vi "USERCallVISample.vi"(4 "Thread No.":u32, 5 "ProgramRef":refnum<vi>, 6 "Thread Mod Recive":refnum<queue>[](array[refnum]), 7 "ThreadsQueue":refnum<queue>[](array[refnum]), 8 "ThreadInfoIN":T1, 10 "StackIn":cluster{"Program":i32, "Prog Index":i32}[](array[cluster]), 11 "PrameterS":string) -> (0 "ThreadInfoOUT":T1, 2 "StackOut":cluster{"Program":i32, "Prog Index":i32}[](array[cluster]), 3 "ErrorCode":string)   [LabVIEW 2019]
panel:
  out "KeyFind?":bool[](array[boolean])
  out "KeyValues":string[](array[string])
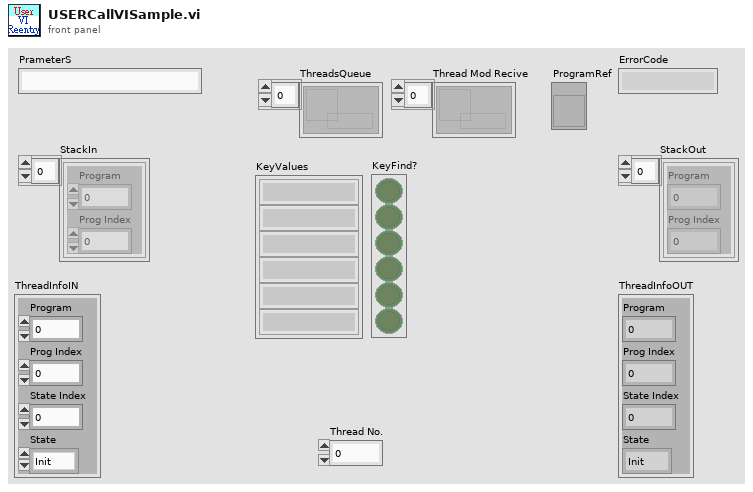
[diagram p1: front panel]
types:
  T1 = cluster{"Program":i32, "Prog Index":i32, "State Index":i32, "State":enum16{"Init", "Idle", "Auto Start", "Auto Running", "Step Start", "Step Running", "Suspend", "Restart", "Stop", "Reset"}}
  T2 = enum16{"Init", "Idle", "Auto Start", "Auto Running", "Step Start", "Step Running", "Suspend", "Restart", "Stop", "Reset"}
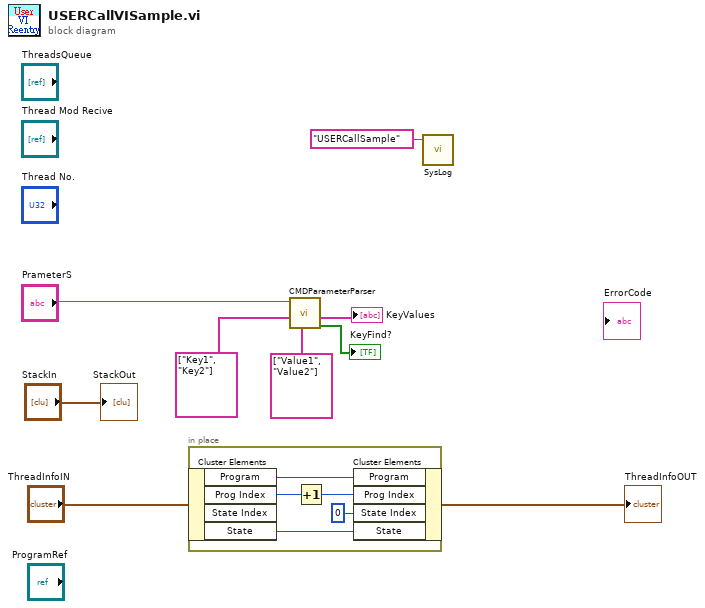
[diagram p0: block diagram]
diagram:
  n1 = in-place {
    n2 = in-place-cluster #1("ThreadInfoIN") -> ("Program"=w14:i32, "Prog Index"=w13:i32, "State"=w10:T2)  [unwired: 1 out]
    n3 = Increment(x=w13) -> (x+1=w12:i32)
    n4 = in-place-cluster #1("Program"=w14, "Prog Index"=w12, "State Index"=0, "State"=w10) -> (→"ThreadInfoOUT":T1)
  }
  n5 = call "CMDParameterParser.vi"("DeafultValues"=string[] ["Value1", "Value2"] ("ParameterKey"), "RequiredKeys"=string[] ["Key1", "Key2"] ("ParameterKey"), "CMDParameter"="PrameterS") -> ("KeyFind?"=→"KeyFind?":bool[], "KeyValues"=→"KeyValues":string[])  [unwired: 6 in, 1 out]
  n6 = call "SysLog.vi"("Mssage"="USERCallSample") -> ()  [unwired: 5 in]
  "StackOut" <- "StackIn"
